vi "Paliwo.vi"() -> ()   [LabVIEW 2017, in "GUI.lvlib"]
uses:
  Libraries/GUI/GUI.lvlib
  Libraries/GUI/Temperatura enum.ctl
panel:
  in  "Array 2":dbl[][](array[numeric])
  out "Color Box 51":u32(colorbox)
  out "Color Box 52":u32(colorbox)
  out "Color Box 53":u32(colorbox)
  out "Color Box 54":u32(colorbox)
  out "Color Box 55":u32(colorbox)
  out "Color Box 56":u32(colorbox)
  out "Color Box 57":u32(colorbox)
  out "Color Box 58":u32(colorbox)
  out "Color Box 59":u32(colorbox)
  out "Color Box 60":u32(colorbox)
  out "Termometr 51":dbl
  out "Termometr 52":dbl
  out "Termometr 53":dbl
  out "Termometr 54":dbl
  out "Termometr 55":dbl
  out "Termometr 56":dbl
  out "Termometr 57":dbl
  out "Termometr 58":dbl
  out "Termometr 59":dbl
  out "Termometr 60":dbl
  out "Color Box 41":u32(colorbox)
  out "Color Box 42":u32(colorbox)
  out "Color Box 43":u32(colorbox)
  out "Color Box 44":u32(colorbox)
  out "Color Box 45":u32(colorbox)
  out "Color Box 46":u32(colorbox)
  out "Color Box 47":u32(colorbox)
  out "Color Box 48":u32(colorbox)
  out "Color Box 49":u32(colorbox)
  out "Color Box 50":u32(colorbox)
  out "Termometr 41":dbl
  out "Termometr 42":dbl
  out "Termometr 43":dbl
  out "Termometr 44":dbl
  out "Termometr 45":dbl
  out "Termometr 46":dbl
  out "Termometr 47":dbl
  out "Termometr 48":dbl
  out "Termometr 49":dbl
  out "Termometr 50":dbl
  out "Color Box 31":u32(colorbox)
  out "Color Box 32":u32(colorbox)
  out "Color Box 33":u32(colorbox)
  out "Color Box 34":u32(colorbox)
  out "Color Box 35":u32(colorbox)
  out "Color Box 36":u32(colorbox)
  out "Color Box 37":u32(colorbox)
  out "Color Box 38":u32(colorbox)
  out "Color Box 39":u32(colorbox)
  out "Color Box 40":u32(colorbox)
  out "Termometr 31":dbl
  out "Termometr 32":dbl
  out "Termometr 33":dbl
  out "Termometr 34":dbl
  out "Termometr 35":dbl
  out "Termometr 36":dbl
  out "Termometr 37":dbl
  out "Termometr 38":dbl
  out "Termometr 39":dbl
  out "Termometr 40":dbl
  out "Color Box 21":u32(colorbox)
  out "Color Box 22":u32(colorbox)
  out "Color Box 23":u32(colorbox)
  out "Color Box 24":u32(colorbox)
  out "Color Box 25":u32(colorbox)
  out "Color Box 26":u32(colorbox)
  out "Color Box 27":u32(colorbox)
  out "Color Box 28":u32(colorbox)
  out "Color Box 29":u32(colorbox)
  out "Color Box 30":u32(colorbox)
  out "Termometr 21":dbl
  out "Termometr 22":dbl
  out "Termometr 23":dbl
  out "Termometr 24":dbl
  out "Termometr 25":dbl
  out "Termometr 26":dbl
  out "Termometr 27":dbl
  out "Termometr 28":dbl
  out "Termometr 29":dbl
  out "Termometr 30":dbl
  out "Color Box 20":u32(colorbox)
  out "Color Box 19":u32(colorbox)
  out "Color Box 18":u32(colorbox)
  out "Color Box 17":u32(colorbox)
  out "Color Box 16":u32(colorbox)
  out "Color Box 15":u32(colorbox)
  out "Color Box 14":u32(colorbox)
  out "Color Box 13":u32(colorbox)
  out "Color Box 12":u32(colorbox)
  out "Color Box 11":u32(colorbox)
  out "Termometr 20":dbl
  out "Termometr 19":dbl
  out "Termometr 18":dbl
  out "Termometr 17":dbl
  out "Termometr 16":dbl
  out "Termometr 15":dbl
  out "Termometr 14":dbl
  out "Termometr 13":dbl
  out "Termometr 12":dbl
  out "Termometr 11":dbl
  out "Color Box 10":u32(colorbox)
  out "Color Box 9":u32(colorbox)
  out "Color Box 8":u32(colorbox)
  out "Color Box 7":u32(colorbox)
  out "Color Box 6":u32(colorbox)
  out "Color Box 5":u32(colorbox)
  out "Color Box 4":u32(colorbox)
  out "Color Box 3":u32(colorbox)
  out "Color Box 2":u32(colorbox)
  out "Color Box":u32(colorbox)
  out "Termometr 10":dbl
  out "Termometr 9":dbl
  out "Termometr 8":dbl
  out "Termometr 7":dbl
  out "Termometr 6":dbl
  out "Termometr 5":dbl
  out "Termometr 4":dbl
  out "Termometr 3":dbl
  out "Termometr 2":dbl
  out "Termometr 1":dbl
  # "STM"
  # "Slave 1"
  # "Slave 2"
  # "Slave 3"
  # "Slave 4"
  # "Slave 5"
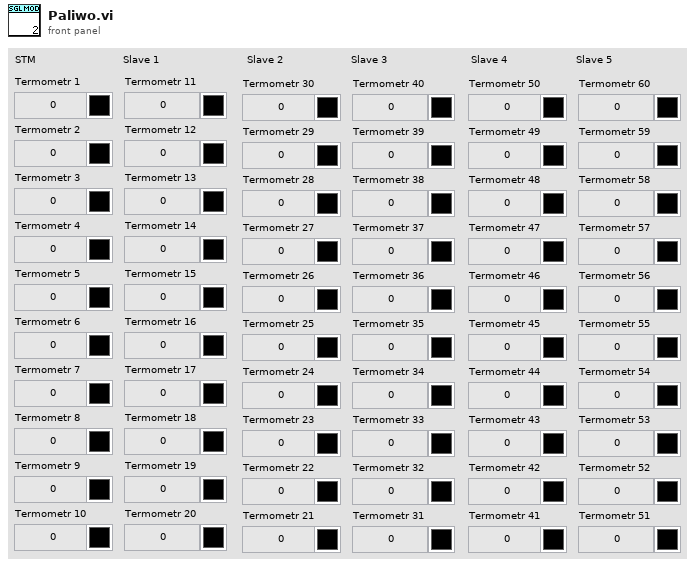
[diagram p1: front panel]
types:
  T1 = typedef "Temperatura enum.ctl" = enum16{"Init", "wait_for_n", "wait_for_data", "S1", "S2", "S3", "S4", "S5", "STM", "Exit"}
  T2 = cluster{"notifier out":refnum<notifier>, "queue out":refnum<queue>}
  T3 = cluster{"PxS":cluster{"Stan Paliwo 1":dbl, "Stan Paliwo 2":dbl, "Stan Paliwo 3":dbl, "Stan Paliwo 4":dbl, "Stan Paliwo 5":dbl, "Stan Paliwo 6":dbl}, bool, "Px":cluster{"Paliwo 1":bool, "Paliwo 2":bool, "Paliwo 3":bool, "Paliwo 4":bool, "Paliwo 5":bool, "Paliwo 6":bool}, "Tx":cluster{"Termometr 1":bool, "Termometr 2":bool, "Termometr 3":bool, "Termometr 4":bool, "Termometr 5":bool, "Termometr 6":bool, "Termometr 7":bool, "Termometr 8":bool, "Termometr 9":bool, "Termometr 10":bool, "Termometr 11":bool, "Termometr 12":bool, "Termometr 13":bool, "Termometr 14":bool, "Termometr 15":bool, "Termometr 16":bool, "Termometr 17":bool, "Termometr 18":bool, "Termometr 19":bool, "Termometr 20":bool}, "TxO":cluster{"T1O":dbl, "T2O":dbl, "T3O":dbl, "T4O":dbl, "T5O":dbl, "T6O":dbl, "T7O":dbl, "T8O":dbl, "T9O":dbl, "T10O":dbl, "T11O":dbl, "T12O":dbl, "T13O":dbl, "T14O":dbl, "T15O":dbl, "T16O":dbl, "T17O":dbl, "T18O":dbl, "T19O":dbl, "T20O":dbl}, "TxA":cluster{"T1A":dbl, "T2A":dbl, "T3A":dbl, "T4A":dbl, "T5A":dbl, "T6A":dbl, "T7A":dbl, "T8A":dbl, "T9A":dbl, "T10A":dbl, "T11A":dbl, "T12A":dbl, "T13A":dbl, "T14A":dbl, "T15A":dbl, "T16A":dbl, "T17A":dbl, "T18A":dbl, "T19A":dbl, "T20A":dbl}}
  T4 = cluster{"output cluster":cluster{"PxS":cluster{"Stan Paliwo 1":dbl, "Stan Paliwo 2":dbl, "Stan Paliwo 3":dbl, "Stan Paliwo 4":dbl, "Stan Paliwo 5":dbl, "Stan Paliwo 6":dbl}, bool, "Px":cluster{"Paliwo 1":bool, "Paliwo 2":bool, "Paliwo 3":bool, "Paliwo 4":bool, "Paliwo 5":bool, "Paliwo 6":bool}, "Tx":cluster{"Termometr 1":bool, "Termometr 2":bool, "Termometr 3":bool, "Termometr 4":bool, "Termometr 5":bool, "Termometr 6":bool, "Termometr 7":bool, "Termometr 8":bool, "Termometr 9":bool, "Termometr 10":bool, "Termometr 11":bool, "Termometr 12":bool, "Termometr 13":bool, "Termometr 14":bool, "Termometr 15":bool, "Termometr 16":bool, "Termometr 17":bool, "Termometr 18":bool, "Termometr 19":bool, "Termometr 20":bool}, "TxO":cluster{"T1O":dbl, "T2O":dbl, "T3O":dbl, "T4O":dbl, "T5O":dbl, "T6O":dbl, "T7O":dbl, "T8O":dbl, "T9O":dbl, "T10O":dbl, "T11O":dbl, "T12O":dbl, "T13O":dbl, "T14O":dbl, "T15O":dbl, "T16O":dbl, "T17O":dbl, "T18O":dbl, "T19O":dbl, "T20O":dbl}, "TxA":cluster{"T1A":dbl, "T2A":dbl, "T3A":dbl, "T4A":dbl, "T5A":dbl, "T6A":dbl, "T7A":dbl, "T8A":dbl, "T9A":dbl, "T10A":dbl, "T11A":dbl, "T12A":dbl, "T13A":dbl, "T14A":dbl, "T15A":dbl, "T16A":dbl, "T17A":dbl, "T18A":dbl, "T19A":dbl, "T20A":dbl}}, cluster{"notifier out":refnum<notifier>, "queue out":refnum<queue>}}
  T5 = cluster{"Array 2[0]":dbl, "Array 2[1]":dbl, "Array 2[2]":dbl, "Array 2[3]":dbl, "Array 2[4]":dbl, "Array 2[5]":dbl, "Array 2[6]":dbl, "Array 2[7]":dbl, "Array 2[8]":dbl, "Array 2[9]":dbl}
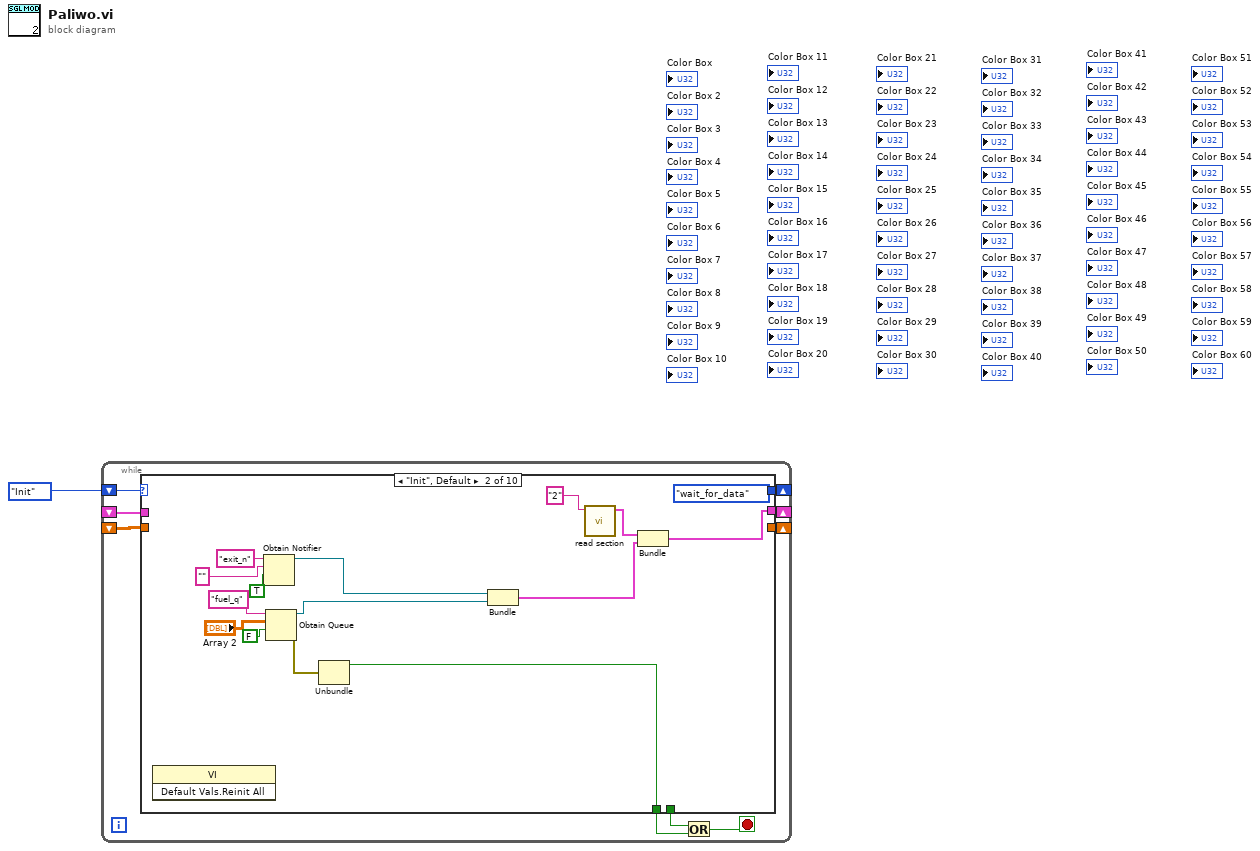
[diagram p0: block diagram]
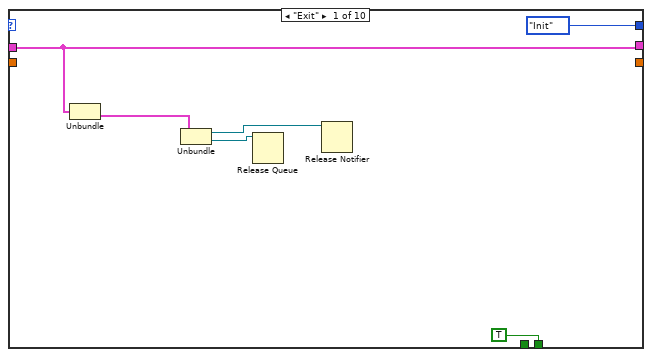
[diagram p2: hidden frame]
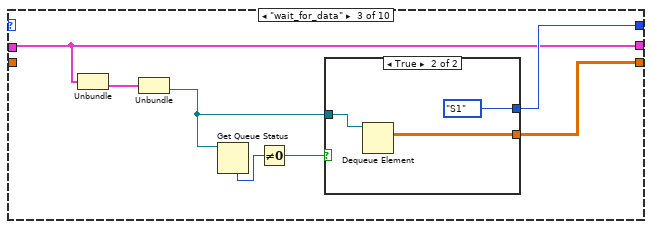
[diagram p3: hidden frame]
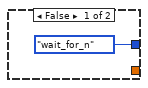
[diagram p4: hidden frame]
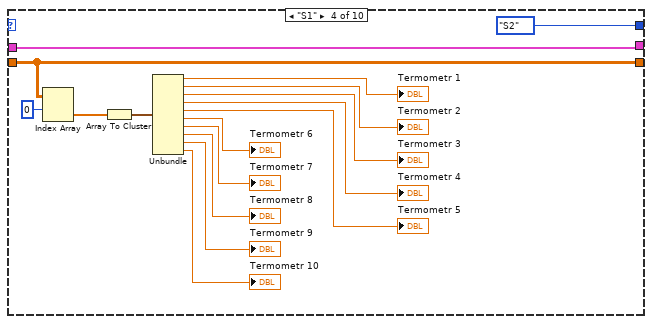
[diagram p5: hidden frame]
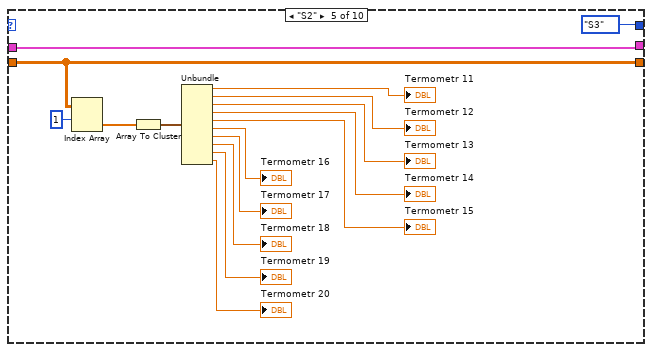
[diagram p6: hidden frame]
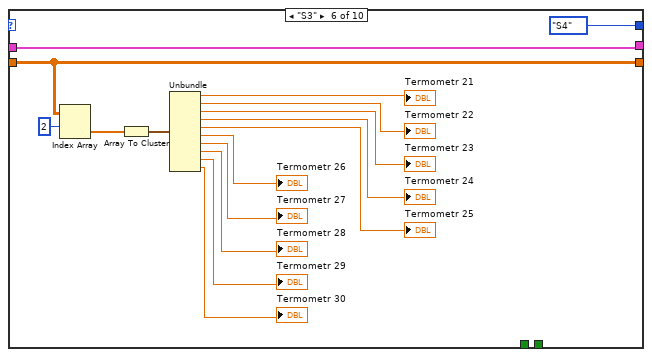
[diagram p7: hidden frame]
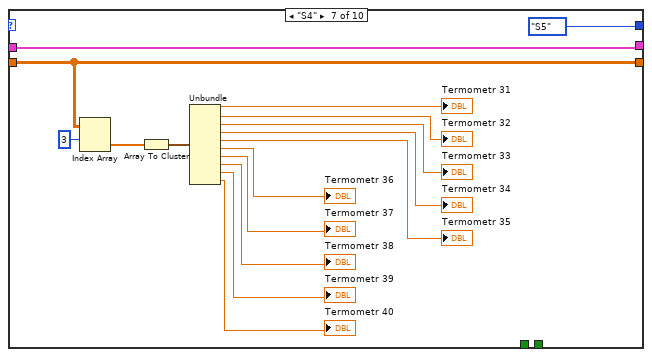
[diagram p8: hidden frame]
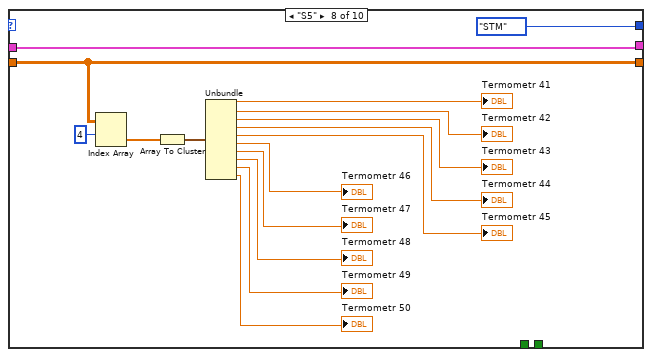
[diagram p9: hidden frame]
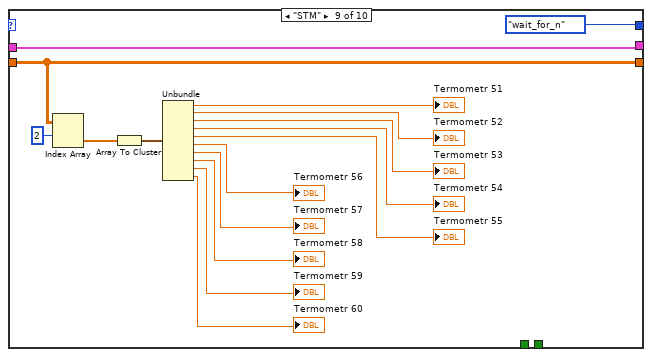
[diagram p10: hidden frame]
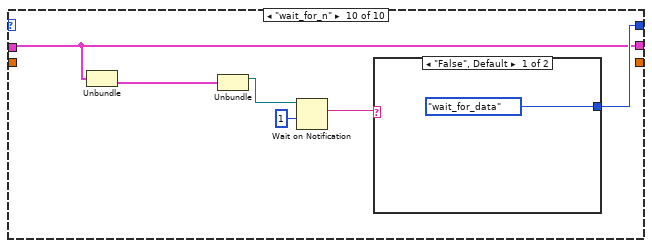
[diagram p11: hidden frame]
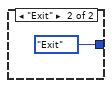
[diagram p12: hidden frame]
diagram:
  n1 = while {
    shift-right: [w7] -> _
    shift-left: _ -> [w6]
    shift-right: [w5] -> _
    shift-left: _ -> [w4]
    shift-right: [w3] -> _
    shift-left: Temperatura_enum."Init" -> [w2]
    stop <- w9 stop-if-true
    n2 = case shown="\"Init\", Default" w2 {
      tunnel: [TRUE _ _ _ _ _ _ _ _ _] -> w8
      tunnel: [_ w27 _ _ _ _ _ _ _ _] -> w10
      tunnel: [Temperatura_enum."Init" Temperatura_enum."wait_for_data" w36 Temperatura_enum."S2" Temperatura_enum."S3" Temperatura_enum."S4" Temperatura_enum."S5" Temperatura_enum."STM" Temperatura_enum."wait_for_n" w144] -> w3
      tunnel: [w12 w20 w33 w57 w73 w89 w105 w121 w137 w140] -> w7
      tunnel: w6 -> [w12 _ w33 w57 w73 w89 w105 w121 w137 w140]
      tunnel: [_ _ w34 w56 w69 w85 w101 w117 w133 _] -> w5
      tunnel: w4 -> [_ _ _ w56 w69 w85 w101 w117 w133 _]
      frame "Exit" {
        n3 = Unbundle(w12) -> (w11:T2)  [unwired: 1 out]
        n4 = Unbundle(w11) -> ("notifier out"=w13:refnum<notifier>, "queue out"=w14:refnum<queue>)
        n5 = Release Queue(queue=w14) -> ()  [unwired: 2 in, 3 out]
        n6 = Release Notifier(notifier=w13) -> ()  [unwired: 2 in, 3 out]
      }
      frame "Init", Default {
        n7 = invoke class="VI" method="Default Vals.Reinit All"() -> ()  [unwired: 3 in, 3 out]
        n8 = Obtain Notifier(name (unnamed)="exit_n", notification data type="", create if not found? (T)=TRUE) -> (notifier out=w24:refnum<notifier>)  [unwired: 1 in, 2 out]
        n9 = Obtain Queue(name (unnamed)="fuel_q", element data type="Array 2", create if not found? (T)=FALSE) -> (queue out=w19:refnum<queue>, error out=w28:errorcluster)  [unwired: 2 in, 1 out]
        n10 = Unbundle(w28) -> ("status"=w27:bool)  [unwired: 2 out]
        n11 = Bundle("notifier out"=w24, "queue out"=w19) -> (w21:T2)  [unwired: 1 in]
        n12 = call "read section.vi"("section"="2") -> ("output cluster"=w17:T3)  [unwired: 10 in]
        n13 = Bundle("output cluster"=w17, w21) -> (w20:T4)  [unwired: 1 in]
      }
      frame "wait_for_data" {
        n14 = Unbundle(w33) -> (w32:T2)  [unwired: 1 out]
        n15 = Unbundle(w32) -> ("queue out"=w35:refnum<queue>)  [unwired: 1 out]
        n16 = Get Queue Status(queue=w35) -> (# elements in queue=w38:i32)  [unwired: 2 in, 7 out]
        n17 = Not Equal To 0?(x=w38) -> (x != 0?=w37:bool)
        n18 = case shown="True" w37 {
          tunnel: [Temperatura_enum."wait_for_n" Temperatura_enum."S1"] -> w36
          tunnel: w35 -> [_ w42]
          tunnel: [_ w40] -> w34
          frame False {
          }
          frame True {
            n19 = Dequeue Element(queue=w42) -> (element=w40:dbl[][])  [unwired: 2 in, 3 out]
          }
        }
      }
      frame "S1" {
        n20 = Index Array(array=w56, index (row)=0) -> (element=w55:dbl[])  [unwired: 1 in]
        n21 = Array To Cluster(array=w55) -> (cluster=w53:T5)
        n22 = Unbundle(w53) -> ("Array 2[0]"=→"Termometr 1":dbl, "Array 2[1]"=→"Termometr 2":dbl, "Array 2[2]"=→"Termometr 3":dbl, "Array 2[3]"=→"Termometr 4":dbl, "Array 2[4]"=→"Termometr 5":dbl, "Array 2[5]"=→"Termometr 6":dbl, "Array 2[6]"=→"Termometr 7":dbl, "Array 2[7]"=→"Termometr 8":dbl, "Array 2[8]"=→"Termometr 9":dbl, "Array 2[9]"=→"Termometr 10":dbl)
      }
      frame "S2" {
        n23 = Index Array(array=w69, index (row)=1) -> (element=w72:dbl[])  [unwired: 1 in]
        n24 = Array To Cluster(array=w72) -> (cluster=w70:T5)
        n25 = Unbundle(w70) -> ("Array 2[0]"=→"Termometr 11":dbl, "Array 2[1]"=→"Termometr 12":dbl, "Array 2[2]"=→"Termometr 13":dbl, "Array 2[3]"=→"Termometr 14":dbl, "Array 2[4]"=→"Termometr 15":dbl, "Array 2[5]"=→"Termometr 16":dbl, "Array 2[6]"=→"Termometr 17":dbl, "Array 2[7]"=→"Termometr 18":dbl, "Array 2[8]"=→"Termometr 19":dbl, "Array 2[9]"=→"Termometr 20":dbl)
      }
      frame "S3" {
        n26 = Index Array(array=w85, index (row)=2) -> (element=w88:dbl[])  [unwired: 1 in]
        n27 = Array To Cluster(array=w88) -> (cluster=w86:T5)
        n28 = Unbundle(w86) -> ("Array 2[0]"=→"Termometr 21":dbl, "Array 2[1]"=→"Termometr 22":dbl, "Array 2[2]"=→"Termometr 23":dbl, "Array 2[3]"=→"Termometr 24":dbl, "Array 2[4]"=→"Termometr 25":dbl, "Array 2[5]"=→"Termometr 26":dbl, "Array 2[6]"=→"Termometr 27":dbl, "Array 2[7]"=→"Termometr 28":dbl, "Array 2[8]"=→"Termometr 29":dbl, "Array 2[9]"=→"Termometr 30":dbl)
      }
      frame "S4" {
        n29 = Index Array(array=w101, index (row)=3) -> (element=w104:dbl[])  [unwired: 1 in]
        n30 = Array To Cluster(array=w104) -> (cluster=w102:T5)
        n31 = Unbundle(w102) -> ("Array 2[0]"=→"Termometr 31":dbl, "Array 2[1]"=→"Termometr 32":dbl, "Array 2[2]"=→"Termometr 33":dbl, "Array 2[3]"=→"Termometr 34":dbl, "Array 2[4]"=→"Termometr 35":dbl, "Array 2[5]"=→"Termometr 36":dbl, "Array 2[6]"=→"Termometr 37":dbl, "Array 2[7]"=→"Termometr 38":dbl, "Array 2[8]"=→"Termometr 39":dbl, "Array 2[9]"=→"Termometr 40":dbl)
      }
      frame "S5" {
        n32 = Index Array(array=w117, index (row)=4) -> (element=w120:dbl[])  [unwired: 1 in]
        n33 = Array To Cluster(array=w120) -> (cluster=w118:T5)
        n34 = Unbundle(w118) -> ("Array 2[0]"=→"Termometr 41":dbl, "Array 2[1]"=→"Termometr 42":dbl, "Array 2[2]"=→"Termometr 43":dbl, "Array 2[3]"=→"Termometr 44":dbl, "Array 2[4]"=→"Termometr 45":dbl, "Array 2[5]"=→"Termometr 46":dbl, "Array 2[6]"=→"Termometr 47":dbl, "Array 2[7]"=→"Termometr 48":dbl, "Array 2[8]"=→"Termometr 49":dbl, "Array 2[9]"=→"Termometr 50":dbl)
      }
      frame "STM" {
        n35 = Index Array(array=w133, index (row)=2) -> (element=w136:dbl[])  [unwired: 1 in]
        n36 = Array To Cluster(array=w136) -> (cluster=w134:T5)
        n37 = Unbundle(w134) -> ("Array 2[0]"=→"Termometr 51":dbl, "Array 2[1]"=→"Termometr 52":dbl, "Array 2[2]"=→"Termometr 53":dbl, "Array 2[3]"=→"Termometr 54":dbl, "Array 2[4]"=→"Termometr 55":dbl, "Array 2[5]"=→"Termometr 56":dbl, "Array 2[6]"=→"Termometr 57":dbl, "Array 2[7]"=→"Termometr 58":dbl, "Array 2[8]"=→"Termometr 59":dbl, "Array 2[9]"=→"Termometr 60":dbl)
      }
      frame "wait_for_n" {
        n38 = Unbundle(w140) -> (w139:T2)  [unwired: 1 out]
        n39 = Unbundle(w139) -> ("notifier out"=w143:refnum<notifier>)  [unwired: 1 out]
        n40 = Wait on Notification(notifier=w143, timeout in ms (-1)=1) -> (notification=w142:string)  [unwired: 2 in, 3 out]
        n41 = case shown="\"False\", Default" w142 {
          tunnel: [Temperatura_enum."wait_for_data" Temperatura_enum."Exit"] -> w144
          frame "False", Default {
          }
          frame "Exit" {
          }
        }
      }
    }
    n42 = Or(x=w8, y=w10) -> (x .or. y?=w9:bool)
  }
